vi "Robot Status.vi"() -> ()   [LabVIEW 2016]
panel:
  out "Robot is in Auto":bool
  out "Flywheel in Long Range Mode":bool
  out "Robot is Turning to Heading":bool
  out "Autoshifting Enabled?":bool
  out "Right Side in Climb Mode?":bool
  out "Robot in High Gear?":bool
  out "Left Side in Climb Mode?":bool
  out "Flywheel at Speed":bool
  out "Robot Has Been Disabled":bool
  out "Robot Has Recently Run Auto":bool
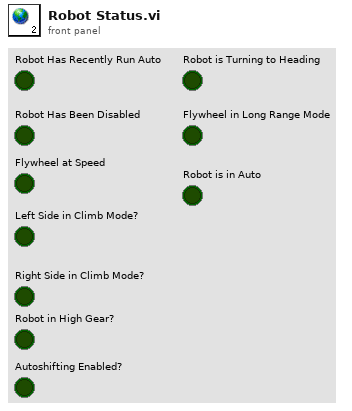
[diagram p1: front panel]
diagram:
